vi "Init SPI.vi"(8 "error in (no error)":errorcluster, 10 "DMA FIFO ref in":refnum<k20>, 11 "Device Ref in":T7 format="%.0x") -> (0 "error out":errorcluster, 2 "DMA FIFO ref out":refnum<k20>, 3 "Compiled Info":T1 {"FIU Engine Data"."Ordered Fault Channels" format="%.0x"; "FIU Engine Data"."FIU IDs"."Slot #" max=15; "FIU Engine Data"."FIU IDs"."Chip Address (A2 A1 A0)" max=7})   [LabVIEW 2014, in "SLSC configuration Engine.lvlib"]
uses:
  SLSC configuration Engine.lvlib
  <vilib>/NI Veristand/Custom Device API/Custom Device Item Ref.ctl
  Shared/SLSC compiled.ctl
  Shared/Res Sim compiled.ctl
  Shared/Type Defs/FIU Engine Data.ctl
  Shared/Type Defs/FIU IDs.ctl
  Example/SPI Utility/Slot #.ctl
  Example/MCP23S17/Chip Address.ctl
  Shared/Constants.vi
  <vilib>/NI Veristand/Custom Device API/Get Item Property (Variant).vi
  <vilib>/Utility/error.llb/Error Cluster From Error Code.vi
  <vilib>/rvi/errors/niLvFpgaAdjustHostInterfaceError.vi
  <vilib>/rvi/interface/nirviMethod/nirviMethod.xnode
  <vilib>/NI Veristand/Custom Device API/Custom Device API.lvlib
  Shared/SLSC configuration Shared.lvlib
  <vilib>/FPGAPlugInAG/Dynamic/niLvFpga_WriteFifo_Dynamic.vi
  <vilib>/rvi/errors/niLvFpgaMergeErrorWithErrorCode.vi
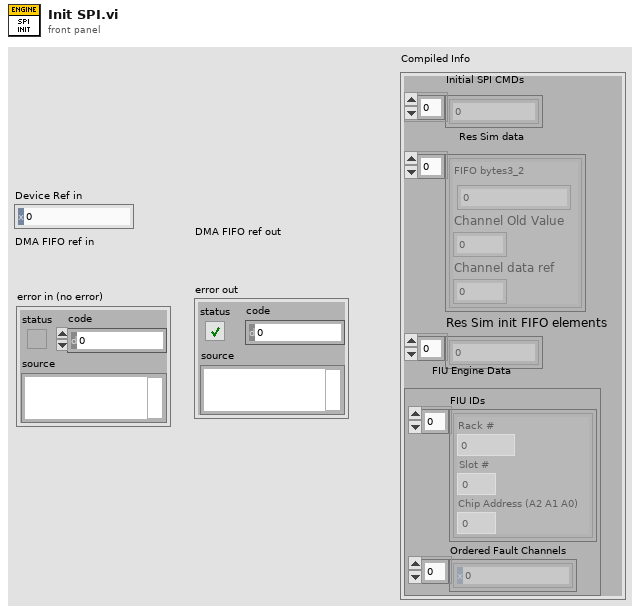
[diagram p1: front panel]
types:
  T1 = typedef "SLSC configuration Shared.lvlib/SLSC compiled.ctl" = cluster{"Initial SPI CMDs":u64[], "Res Sim data ":T2[], "Res Sim init FIFO elements":u32[], "FIU Engine Data":T3}
  T2 = typedef "SLSC configuration Shared.lvlib/Res Sim compiled.ctl" = cluster{"FIFO bytes3_2":u16, "Channel Old Value":dbl, "Channel data ref":i32}
  T3 = typedef "SLSC configuration Shared.lvlib/FIU Engine Data.ctl" = cluster{"FIU IDs":T4[], "Ordered Fault Channels":T7[]}
  T4 = typedef "SLSC configuration Shared.lvlib/FIU IDs.ctl" = cluster{"Rack #":u8, "Slot #":T5, "Chip Address (A2 A1 A0)":T6}
  T5 = typedef "SLSC configuration Shared.lvlib/Slot #.ctl" = u8
  T6 = typedef "SLSC configuration Shared.lvlib/Chip Address.ctl" = u8
  T7 = typedef "Custom Device API.lvlib/Custom Device Item Ref.ctl" = u64
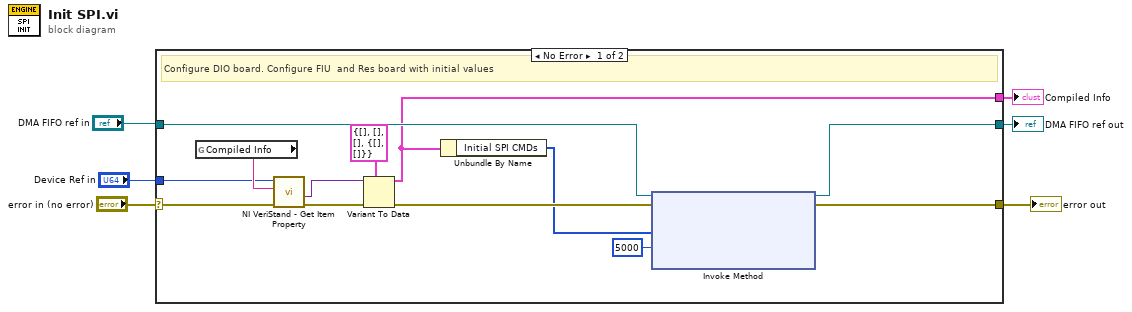
[diagram p0: block diagram]
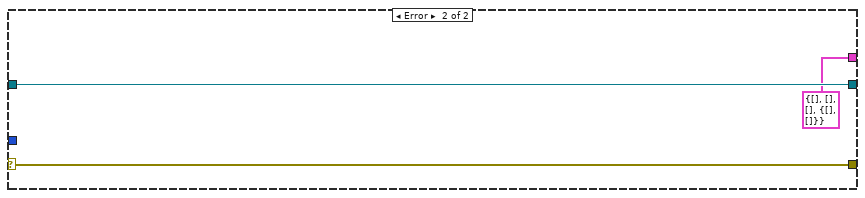
[diagram p2: hidden frame]
diagram:
  n1 = case shown="No Error" "error in (no error)" {
    selector: "error in (no error)" -> [w10 w21]
    tunnel: "DMA FIFO ref in" -> [w14 w22]
    tunnel: [w12 w22] -> w1
    tunnel: [w8 w21] -> w6
    tunnel: "Device Ref in" -> [w11 _]
    tunnel: [w9 T1 {"Initial SPI CMDs"=[], "Res Sim data "=[], "Res Sim init FIFO elements"=[], "FIU Engine Data"={"FIU IDs"=[], "Ordered Fault Channels"=[]}} ("type")] -> w3
    frame No Error {
      # "Configure DIO board. Configure FIU  and Res board with initial values"
      n2 = global read "Constants.vi" "Compiled Info"() -> (w19:string)
      n3 = call-poly <vilib>:"NI VeriStand - Get Item Property.vi"("error in (no error)"=w10, "Property Name"=w19, "Item Ref in"=w11) -> ("error out"=w18:errorcluster, "Value"=w17:variant)  [unwired: 5 in, 2 out]
      n4 = Variant To Data(error in=w18, type=T1 {"Initial SPI CMDs"=[], "Res Sim data "=[], "Res Sim init FIFO elements"=[], "FIU Engine Data"={"FIU IDs"=[], "Ordered Fault Channels"=[]}}, Variant=w17) -> (data=w9:T1, error out=w15:errorcluster)
      n5 = Unbundle By Name(w9) -> ("Initial SPI CMDs"=w7:u64[])
      n6 = xnode "Invoke Method"("FPGA VI Reference In"=w14, "error in"=w15, "Data"=w7, "Timeout (ms)"=5000) -> ("FPGA VI Reference Out"=w12:refnum<k20>, "error out"=w8:errorcluster)  [unwired: 1 out]
    }
    frame Error {
    }
  }
  "error out" <- w6
  "Compiled Info" <- w3
  "DMA FIFO ref out" <- w1
